vi "Read Sessions.vi"(11 "TCPConnectionHandler in":refnum<class "TCPConnectionHandler.lvclass">) -> (2 "Sessions":refnum<class "Session.lvclass">[](array[class]), 3 "TCPConnectionHandler out":refnum<class "TCPConnectionHandler.lvclass">)   [LabVIEW 2013, in "MQTT_TCP.lvlib" / "TCPConnectionHandler.lvclass"]
uses:
  TCPConnectionHandler.lvclass
  MQTT_Base/Session/Session.lvclass
  TCPConnectionHandler.lvclass/TCPConnectionHandler.ctl
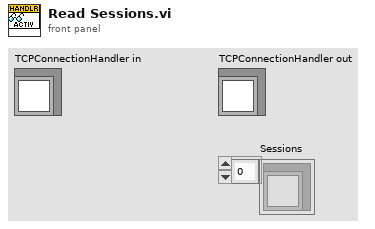
[diagram p1: front panel]
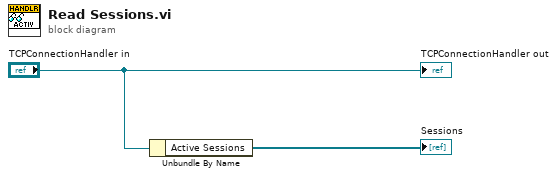
[diagram p0: block diagram]
diagram:
  n1 = Unbundle By Name("TCPConnectionHandler in") -> ("Active Sessions"=→"Sessions":refnum<class "Session.lvclass">[])
  "TCPConnectionHandler out" <- "TCPConnectionHandler in"
